vi "Zero Phase Lowpass Filter (single).vi"(8 "error in (no error)":errorcluster, 10 "cutoff period":dbl, 11 "XY-data":cluster{"X-array":dbl[], "Y-array":dbl[]}) -> (0 "error out":errorcluster, 3 "XY-data out":cluster{"X-array":dbl[], "Y-array":dbl[]} {"Y-array" format="%.2p"; "X-array" format="%.2p"})   [LabVIEW 2019, in "xy_utilities.lvlib"]
doc: "Apply a Zero Phase Lowpass Filter to <b>XY-Data<b/>'s Y-Array.\n\n<b>cutoff period</b> is equivalent to 1/cutoff frequency and is in the units of the X-Array. The cutoff frequency is restricted between 0 and Fs/4.\n\nWire data to the data input to determine the polymorphic instance to use or manually select the instance."
uses:
  xy_utilities.lvlib
  <vilib>/Analysis/3filter.llb/Filter Passband Type.ctl
  <vilib>/Analysis/NI_AALBase.lvlib
  <vilib>/Analysis/3filter.llb/Zero Phase Filter (DBL).vi
  <vilib>/Analysis/4window.llb/windowTd.ctl
  <vilib>/Analysis/NI_AALPro.lvlib
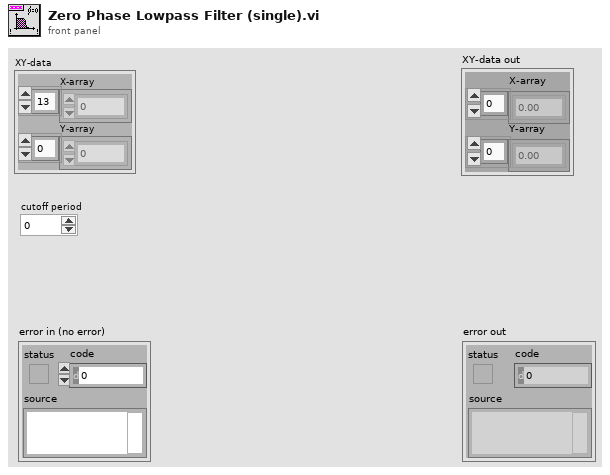
[diagram p1: front panel]
types:
  T1 = typedef "NI_AALBase.lvlib/Filter Passband Type.ctl" = enum32{"Lowpass", "Highpass", "Bandpass", "Bandstop"}
  T2 = typedef "NI_AALPro.lvlib/windowTd.ctl" = u32
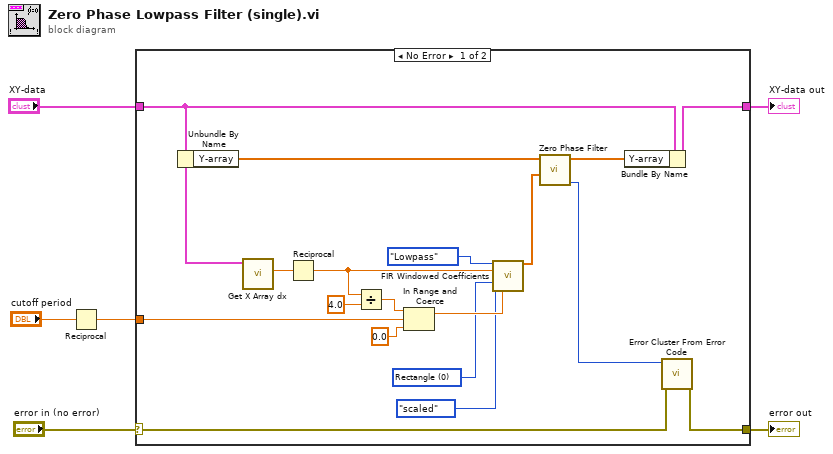
[diagram p0: block diagram]
diagram:
  n1 = Reciprocal(x="cutoff period") -> (1/x=w2:dbl)
  n2 = case shown="No Error" "error in (no error)" {
    selector: "error in (no error)" -> [w23 w26]
    tunnel: [w22 w26] -> w5
    tunnel: "XY-data" -> [w9 w25]
    tunnel: [w24 w25] -> w3
    tunnel: w2 -> [w18 _]
    frame No Error {
      w14 = T2 0 items=["Rectangle"=0, "Hanning"=1, "Hamming"=2, "Blackman-Harris"=3, "Exact Blackman"=4, "Blackman"=5, "Flat Top"=6, "4 Term B-Harris "=7, "7 Term B-Harris"=8, "Low Sidelobe"=9, "Blackman Nuttall"=11, "Triangle"=30, "Bartlett-Hanning"=31, "Bohman"=32, "Parzen"=33, "Welch"=34, "Kaiser"=60, "Dolph-Chebyshev"=61, "Gaussian"=62] ("window")
      n3 = Unbundle By Name(w9) -> ("Y-array"=w21:dbl[])
      n4 = call "Get X Array dx.vi"("XY-data"=w9) -> ("dX"=w8:dbl)  [unwired: 7 in, 3 out]
      n5 = Reciprocal(x=w8) -> (1/x=w7:dbl)
      n6 = Divide(x=w7, y=4.0) -> (x/y=w20:dbl)
      n7 = In Range and Coerce(upper limit=w20, x=w18, lower limit=0.0) -> (coerced(x)=w15:dbl)  [unwired: 1 out]
      n8 = call <vilib>:"FIR Windowed Coefficients.vi"("filter type"=Filter_Passband_Type."Lowpass", "sampling freq: fs"=w7, "window"=w14, "option"=enum32{"not scaled", "scaled"}."scaled", "low cutoff freq: fl"=w15) -> ("FIR Windowed Coefficients"=w12:dbl[])  [unwired: 9 in, 1 out]
      n9 = call-poly <vilib>:"Zero Phase Filter.vi"("Forward Coefficients"=w12, "X"=w21) -> ("error"=w11:i32, "Filtered X"=w16:dbl[])  [unwired: 8 in]
      n10 = Bundle By Name(cluster=w9, "Y-array"=w16) -> (w24:cluster{"X-array":dbl[], "Y-array":dbl[]})
      n11 = call <vilib>:"Error Cluster From Error Code.vi"("error in (no error)"=w23, "error code (0)"=w11) -> ("error out"=w22:errorcluster)  [unwired: 7 in]
    }
    frame Error {
    }
  }
  "error out" <- w5
  "XY-data out" <- w3
